vi "Create.vi"(8 "error in (no error)":errorcluster, 10 "Test Tree reference":refnum<vi>) -> (0 "error out":errorcluster, 3 "Test Result Tree V2 out":refnum<class "Test Result Tree V2.lvclass">)   [LabVIEW 2020, in "Test Result Tree V2.lvclass"]
uses:
  Test Result Tree V2.lvclass
  Test Result Tree V2.lvclass/Test Result Tree V2.ctl
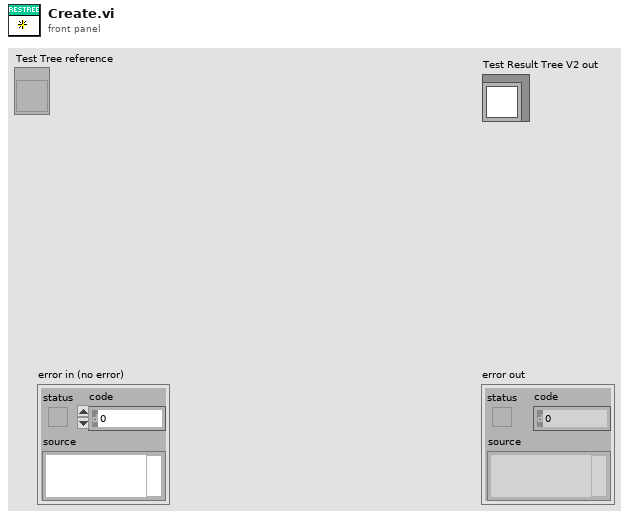
[diagram p1: front panel]
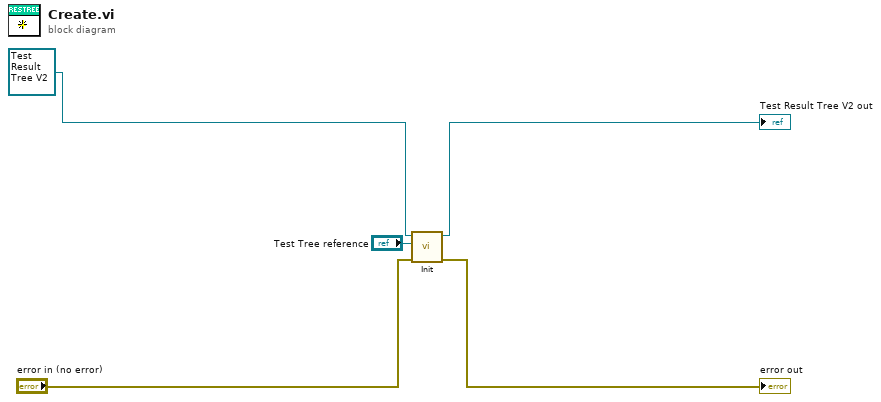
[diagram p0: block diagram]
diagram:
  n1 = call-dynamic "Init.vi"("error in (no error)"="error in (no error)", "Test Tree reference"="Test Tree reference", "Test Tree In"=refnum<class "Test Result Tree V2.lvclass"> refnum ("Test Result Tree V2 in")) -> ("error out"=→"error out":errorcluster, "Test Tree Out"=→"Test Result Tree V2 out":refnum<class "Test Result Tree V2.lvclass">)  [unwired: 7 in]
